vi "IMAQdx Grab.vi"(8 "error in":errorcluster, 9 "Wait for Next Buffer? (Yes)":bool=TRUE, 10 "Image In":T2, 11 "Session In":T1) -> (0 "error out":errorcluster, 1 "Buffer Number Out":u32, 2 "Image Out":T2, 3 "Session Out":T1)   [LabVIEW 2013, in "NI_Vision_Acquisition_Software.lvlib"]
doc: "Acquires the most current frame into Image Out. Call this VI only after calling IMAQdx Configure Grab.vi. If the image type does not match the video format of the camera, this VI changes the image type to a suitable format."
uses:
  NI_Vision_Acquisition_Software.lvlib
  IMAQdx.ctl
  IMAQ Image.ctl
  IMAQdx Buffer Number Mode.ctl
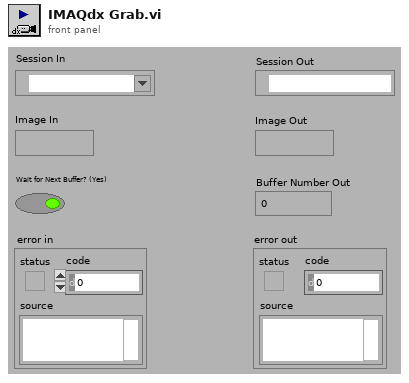
[diagram p1: front panel]
types:
  T1 = typedef "IMAQdx.ctl" = refnum<k21>
  T2 = typedef "IMAQ Image.ctl" = refnum<image>
  T3 = typedef "NI_Vision_Acquisition_Software.lvlib/IMAQdx Buffer Number Mode.ctl" = enum32{"Next", "Last", "Buffer Number"}
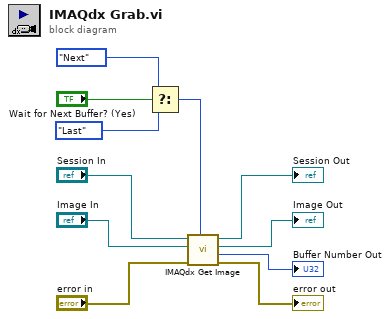
[diagram p0: block diagram]
diagram:
  n1 = Select(t=IMAQdx_Buffer_Number_Mode."Next" ("Buffer Number Mode"), s="Wait for Next Buffer? (Yes)", f=IMAQdx_Buffer_Number_Mode."Last" ("Buffer Number Mode")) -> (s? t:f=w2:T3)
  n2 = call "IMAQdx Get Image.vi"("Buffer Number Mode (Next)"=w2, "error in"="error in", "Image In"="Image In", "Session In"="Session In") -> ("error out"=→"error out":errorcluster, "Buffer Number Out"=→"Buffer Number Out":u32, "Image Out"=→"Image Out":T2, "Session Out"=→"Session Out":T1)  [unwired: 4 in]
